vi "Read Gueret Prins Instances.vi"(8 "error in (no error)":errorcluster, 11 "OSSP_Problem in":refnum<class "OSSP_Problem.lvclass">) -> (0 "error out":errorcluster, 3 "OSSP_Problem out":refnum<class "OSSP_Problem.lvclass">)   [LabVIEW 2013, in "OSSP_Problem.lvclass"]
uses:
  OSSP_Problem.lvclass
  OSSP_Problem.lvclass/OSSP_Problem.ctl
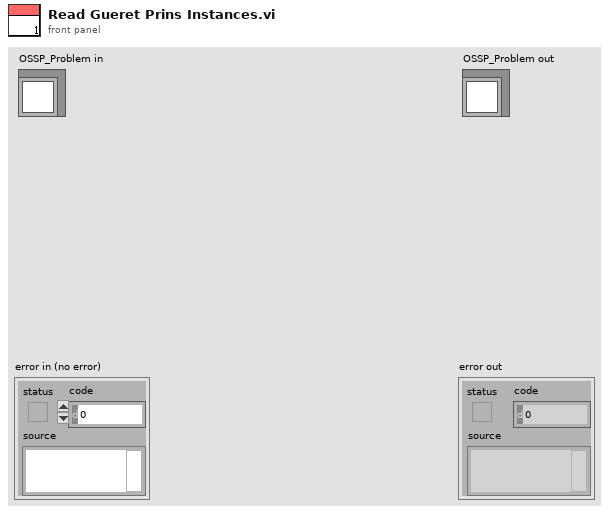
[diagram p1: front panel]
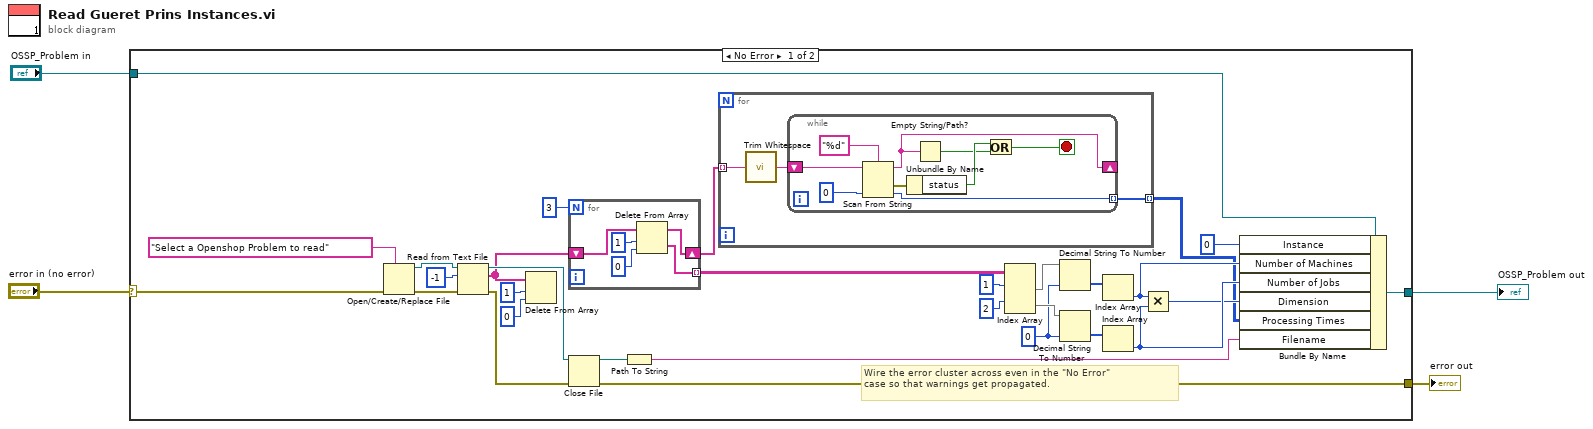
[diagram p0: block diagram]
diagram:
  n1 = case shown="No Error" "error in (no error)" {
    selector: "error in (no error)" -> [w16 w53]
    tunnel: [w15 w53] -> w3
    tunnel: [w12 w52] -> w1
    tunnel: "OSSP_Problem in" -> [w13 w52]
    frame No Error {
      w18 = u8 0 ("default (0 I32)")
      # "Wire the error cluster across even in the \"No Error\"\ncase so that warnings get propagated."
      n2 = Open/Create/Replace File(error in=w16, prompt="Select a Openshop Problem to read") -> (refnum out=w7:refnum<file>, error out=w30:errorcluster)  [unwired: 4 in, 1 out]
      n3 = Read from Text File(file (use dialog)=w7, count=-1, error in=w30) -> (refnum out=w32:refnum<file>, text=w26:string[], error out=w31:errorcluster)  [unwired: 1 in, 1 out]
      n4 = Delete From Array(array=w26, length=1 ("index"), index=0) -> ()  [unwired: 2 out]
      n5 = for {
        N: 3 -> [_]
        shift-right: [w50] -> w17
        shift-left: w26 -> [w51]
        tunnel: [w49] -> w25 mode=indexing
        n6 = Delete From Array(array=w51, length=1, index=0) -> (deleted portion=w49:string[], array with subset deleted=w50:string[])
      }
      n7 = Close File(refnum=w32, error in=w31) -> (path=w6:path, error out=w15:errorcluster)
      n8 = Path To String(path=w6) -> (string=w5:string)
      n9 = for {
        tunnel: w17 -> [w36] mode=indexing
        tunnel: [w37] -> w8 mode=indexing
        n10 = call <vilib>:"Trim Whitespace.vi"("string"=w36) -> ("trimmed string"=w35:string)  [unwired: 1 in]
        n11 = while {
          shift-right: [w42] -> _
          shift-left: w35 -> [w46]
          tunnel: [w44] -> w37 mode=indexing
          stop <- w38 stop-if-true
          n12 = Scan From String(format string="%d", input string=w46, default 1=u16 0 ("default value 1")) -> (remaining string=w42:string, error out=w41:errorcluster, output 1=w44:u16)  [unwired: 2 in, 1 out]
          n13 = Unbundle By Name(w41) -> ("status"=w40:bool)
          n14 = Empty String/Path?(string/path=w42) -> (empty?=w39:bool)
          n15 = Or(x=w40, y=w39) -> (x .or. y?=w38:bool)
        }
      }
      n16 = Index Array(array=w25, index (row) #1=1 ("index"), index (row) #2=2 ("index")) -> (element #1=w22:string[], element #2=w21:string[])  [unwired: 2 in]
      n17 = Decimal String To Number(string=w22, default (0L)=w18) -> (number=w20:u8[])  [unwired: 1 in, 1 out]
      n18 = Decimal String To Number(string=w21, default (0L)=w18) -> (number=w19:u8[])  [unwired: 1 in, 1 out]
      n19 = Index Array(array=w20) -> (element=w11:u8)  [unwired: 1 in]
      n20 = Index Array(array=w19) -> (element=w10:u8)  [unwired: 1 in]
      n21 = Multiply(x=w11, y=w10) -> (x*y=w9:u8)
      n22 = Bundle By Name(cluster=w13, "Instance"=u8 0, "Number of Machines"=w11, "Number of Jobs"=w10, "Dimension"=w9, "Processing Times"=w8, "Filename"=w5) -> (w12:refnum<class "OSSP_Problem.lvclass">)
    }
    frame Error {
    }
  }
  "error out" <- w3
  "OSSP_Problem out" <- w1
